vi "UIWriteCtrlCluster.vi"(7 "Class_Hierarchy (F)":bool, 8 "error in":errorcluster, 9 "Control Value":variant, 10 "callerName":string) -> (0 "error out":errorcluster, 1 "NestedCtrlValues":variant[](array[variant]), 2 "NestedCtrlNames":string[](array[string]))   [LabVIEW 2025, in "UI_Library.lvlib" / "UI_Library.lvclass"]
doc: "Get Cluster sub Controls name and value recursively"
uses:
  UI_Library.lvclass
  <vilib>/Utility/Data Type/NI_Data Type.lvlib
  <vilib>/PNR/LabVIEW Composition/Composition/Composition.lvlib
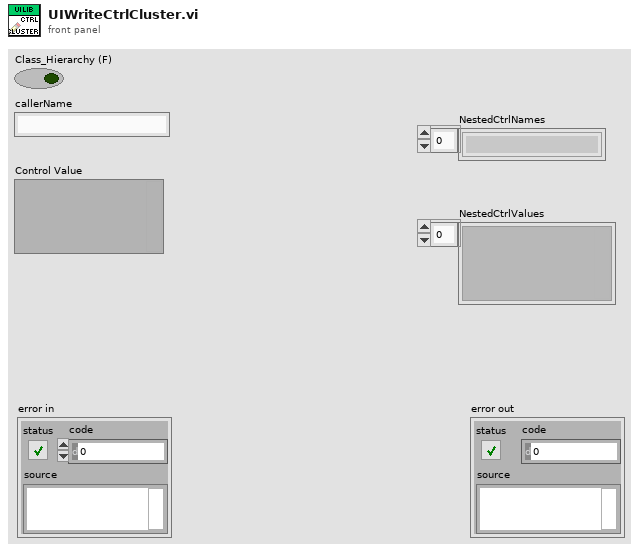
[diagram p1: front panel]
types:
  T1 = typedef "NI_Data Type.lvlib/Data Type.ctl" = enum8{"Invalid Type", "Void", "I8", "I16", "I32", "I64", "U8", "U16", "U32", "U64", "Single Float", "Double Float", "Extended Float", "Single Complex", "Double Complex", "Extended Complex", "Enum U8", "Enum U16", "Enum U32", "Enum U64", "Single Float With Unit", "Double Float With Unit", "Extended Float With Unit", "Single Complex with Unit", "Double Complex with Unit", "Extended Complex with Unit", "Boolean", "String", "Path", "Picture", "Tag", "Array", "Cluster", "Variant", "LV Variant", "Waveform", "Timestamp", "Digital Waveform", "Digital Data", "ExpressData", "Refnum", "External Data", "VI", "Poly VI", "LabVIEW Class Instance", "Fixed Point", "Set Collection", "Map Collection"}
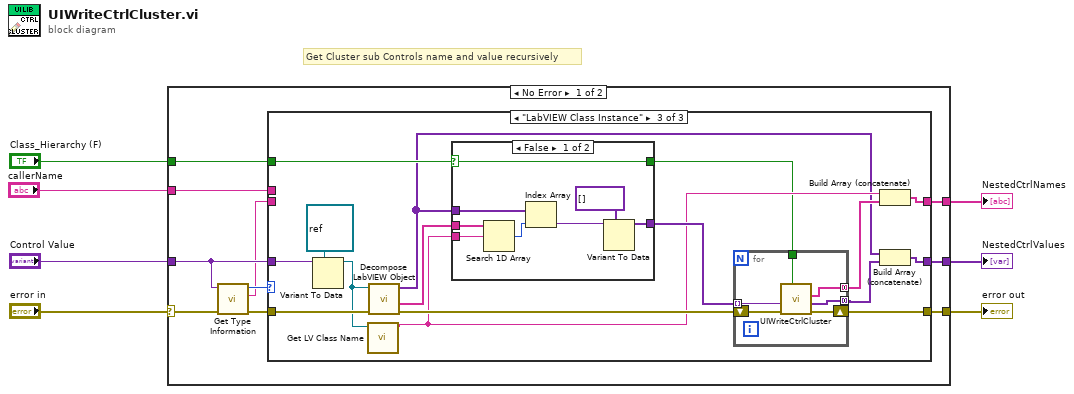
[diagram p0: block diagram]
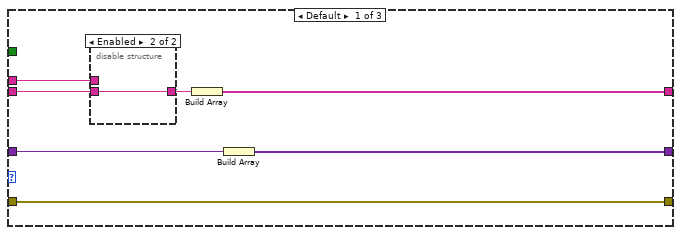
[diagram p2: hidden frame]
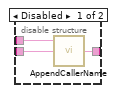
[diagram p3: hidden frame]
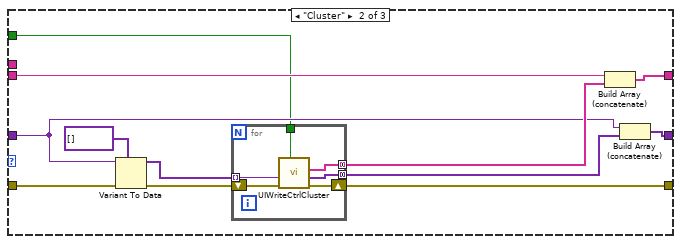
[diagram p4: hidden frame]
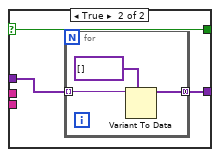
[diagram p5: hidden frame]
diagram:
  # "Get Cluster sub Controls name and value recursively"
  n1 = case shown="No Error" "error in" {
    selector: "error in" -> [w17 w83]
    tunnel: [w12 w83] -> w7
    tunnel: "Control Value" -> [w14 _]
    tunnel: [w11 _] -> w4
    tunnel: [w9 _] -> w3
    tunnel: "callerName" -> [w10 _]
    tunnel: "Class_Hierarchy (F)" -> [w8 _]
    frame No Error {
      n2 = call <vilib>:"Get Type Information.vi"("error in (no error)"=w17, "variant"=w14) -> ("error out"=w16:errorcluster, "name"=w13:string, "type"=w15:T1)  [unwired: 5 in, 2 out]
      n3 = case shown="\"LabVIEW Class Instance\"" w15 {
        tunnel: w16 -> [w21 w39 w61]
        tunnel: w14 -> [w24 w30 w55]
        tunnel: [w23 w32 w51] -> w11
        tunnel: [w22 w33 w50] -> w9
        tunnel: w13 -> [w20 w31 _]
        tunnel: [w21 w37 w58] -> w12
        tunnel: w10 -> [w18 _ _]
        tunnel: w8 -> [_ w29 w52]
        frame Default {
          n4 = disable-structure "Diagram Disable Structure" shown="Enabled" {
            disable-tunnel: w20 -> [w27 w28]
            disable-tunnel: [w26 w28] -> w19
            disable-tunnel: w18 -> [w25 _]
            frame Disabled {
              n5 = call "AppendCallerName.vi"("B"=w27, "A"=w25) -> ("A.B"=w26:string)  [unwired: 1 in]
            }
            frame Enabled {
            }
          }
          n6 = Build Array(w19) -> (w22:string[])
          n7 = Build Array(w24) -> (w23:variant[])
        }
        frame "Cluster" {
          n8 = Variant To Data(error in=w39, type=variant[] [], Variant=w30) -> (data=w36:variant[], error out=w38:errorcluster)
          n9 = for {
            tunnel: w36 -> [w44] mode=indexing
            tunnel: [w43] -> w35 mode=concatenating
            tunnel: [w42] -> w34 mode=concatenating
            shift-right: [w45] -> w37
            shift-left: w38 -> [w46]
            tunnel: w29 -> [w41]
            n10 = call "UIWriteCtrlCluster.vi"("Class_Hierarchy (F)"=w41, "error in"=w46, "Control Value"=w44) -> ("error out"=w45:errorcluster, "NestedCtrlValues"=w42:variant[], "NestedCtrlNames"=w43:string[])  [unwired: 6 in]
          }
          n11 = Build Array (concatenate)(w31, w35) -> (w33:string[])
          n12 = Build Array (concatenate)(w30, w34) -> (w32:variant[])
        }
        frame "LabVIEW Class Instance" {
          n13 = Variant To Data(type=refnum<class> refnum ("LabVIEW Object"), Variant=w55) -> (data=w54:refnum<class>)  [unwired: 1 in, 1 out]
          n14 = call <vilib>:"Get LV Class Name.vi"("object"=w54) -> ("class name"=w49:string)  [unwired: 9 in, 1 out]
          n15 = call <vilib>:"Decompose LabVIEW Object.vi"("error in (no error)"=w61, "LabVIEW Object"=w54) -> ("error out"=w60:errorcluster, "Class Names"=w53:string[], "Private Data Clusters"=w48:variant[])  [unwired: 6 in, 1 out]
          n16 = case shown="False" w52 {
            selector: w52 -> [w63 w71]
            tunnel: w48 -> [w68 w73]
            tunnel: [w70 w72] -> w59
            tunnel: w53 -> [w66 _]
            tunnel: w49 -> [w65 _]
            tunnel: [w63 w71] -> w47
            frame False {
              n17 = Search 1D Array(1D array=w66, element=w65) -> (index of element=w67:i32)  [unwired: 1 in]
              n18 = Index Array(array=w68, index=w67) -> (element=w69:variant)
              n19 = Variant To Data(type=variant[] [], Variant=w69) -> (data=w70:variant[])  [unwired: 1 in, 1 out]
            }
            frame True {
              n20 = for {
                tunnel: w73 -> [w75] mode=indexing
                tunnel: [w74] -> w72 mode=concatenating
                n21 = Variant To Data(type=variant[] [], Variant=w75) -> (data=w74:variant[])  [unwired: 1 in, 1 out]
              }
            }
          }
          n22 = for {
            tunnel: w59 -> [w80] mode=indexing
            tunnel: [w79] -> w56 mode=concatenating
            tunnel: [w78] -> w57 mode=concatenating
            shift-right: [w81] -> w58
            shift-left: w60 -> [w82]
            tunnel: w47 -> [w77]
            n23 = call "UIWriteCtrlCluster.vi"("Class_Hierarchy (F)"=w77, "error in"=w82, "Control Value"=w80) -> ("error out"=w81:errorcluster, "NestedCtrlValues"=w78:variant[], "NestedCtrlNames"=w79:string[])  [unwired: 6 in]
          }
          n24 = Build Array (concatenate)(w49, w56) -> (w50:string[])
          n25 = Build Array (concatenate)(w48, w57) -> (w51:variant[])
        }
      }
    }
    frame Error {
    }
  }
  "error out" <- w7
  "NestedCtrlValues" <- w4
  "NestedCtrlNames" <- w3
